vi "2.feladat.vi"() -> ()   [LabVIEW 2015]
panel:
  in  "m/s":dbl
  out "?":dbl
  out "Boolean 2":bool
  in  "Boolean":bool
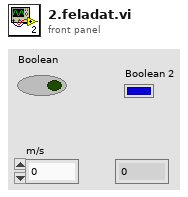
[diagram p1: front panel]
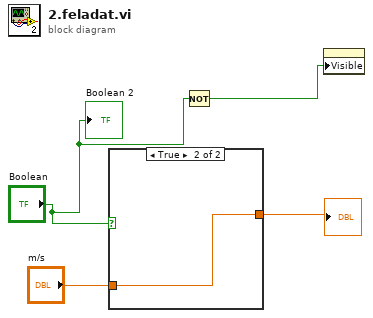
[diagram p0: block diagram]
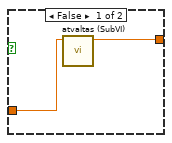
[diagram p2: hidden frame]
diagram:
  n1 = case shown="True" "Boolean" {
    tunnel: "m/s" -> [w6 w7]
    tunnel: [w5 w7] -> w3
    frame False {
      n2 = call "atvaltas (SubVI).vi"("m/s"=w6) -> ("km/h"=w5:dbl)  [unwired: 10 in]
    }
    frame True {
    }
  }
  "?" <- w3
  n3 = Not(x="Boolean") -> (.not. x?=w1:bool)
  n4 = property class="DigNum (strict)"("Visible"=w1) -> ()  [unwired: 2 in, 2 out]
  "Boolean 2" <- "Boolean"
